vi "Scale min and max.vi"(2 "Display Type":enum16{"X", "Y", "MAG", "PHASE"}(ring), 3 "Sensitivity String":string) -> (0 "Scale.Range:Minimum":dbl, 1 "Scale.Range:Maximum":dbl)   [LabVIEW 2016, in "Instrument.SR7270 UI.lvclass"]
uses:
  Instrument.SR7270 UI.lvclass
  Instrument.SR7270/Driver/SR7270 Drivers.lvlib
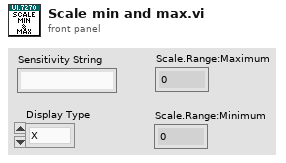
[diagram p1: front panel]
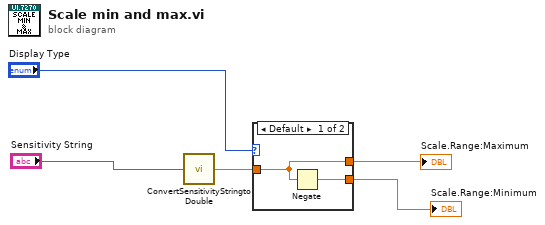
[diagram p0: block diagram]
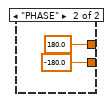
[diagram p2: hidden frame]
diagram:
  n1 = call "ConvertSensitivityStringtoDouble.vi"("Sensitivity"="Sensitivity String") -> ("Sensitivtiy"=w1:dbl)
  n2 = case shown="Default" "Display Type" {
    tunnel: [w7 180.0 ("Scale.Range:Maximum")] -> w5
    tunnel: [w6 -180.0 ("Scale.Range:Maximum")] -> w4
    tunnel: w1 -> [w7 _]
    frame Default {
      n3 = Negate(x=w7) -> (-x=w6:dbl)
    }
    frame "PHASE" {
    }
  }
  "Scale.Range:Maximum" <- w5
  "Scale.Range:Minimum" <- w4
